vi "test.vi"() -> ()   [LabVIEW 2010]
uses:
  XIntensityCompensation.xctl
panel:
  in  "free-run mode?":bool
  in  "stop":bool
  in  "XIntensityCompensation":cluster{"A":dbl, "lambda":dbl[unit], "C":dbl}(xcontrol)
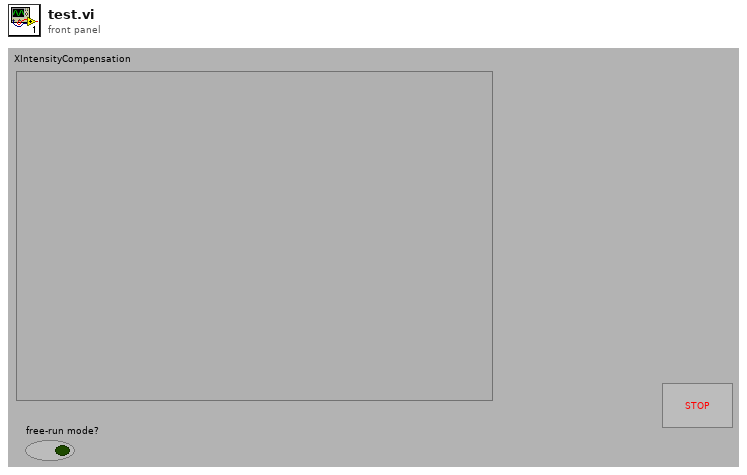
[diagram p1: front panel]
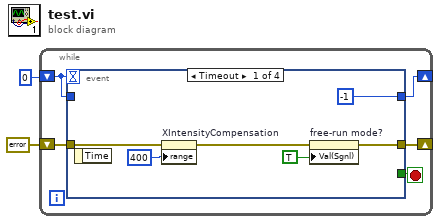
[diagram p0: block diagram]
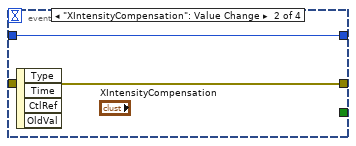
[diagram p2: hidden frame]
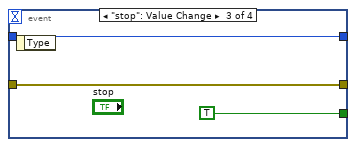
[diagram p3: hidden frame]
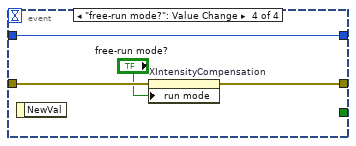
[diagram p4: hidden frame]
diagram:
  n1 = while {
    shift-right: [w5] -> _
    shift-left: errorcluster {"status"=FALSE, "code"=0, "source"=""} ("error in (no error)") -> [w6]
    shift-right: [w3] -> _
    shift-left: 0 -> [w4]
    stop <- w7 stop-if-true
    n2 = event shown="[0] Timeout" {
      selector: _ -> [_ _ _ _]
      dyn-events: _ -> [_ _ _ _]
      timeout: w4 -> [_ _ _ _]
      tunnel: [_ _ TRUE _] -> w7
      tunnel: w6 -> [w10 w15 w17 w22]
      tunnel: [w12 w15 w17 w21] -> w5
      tunnel: w4 -> [_ w14 w16 w20]
      tunnel: [-1 w14 w16 w20] -> w3
      event Timeout {
        n3 = event-data() -> ()  [unwired: 1 in, 1 out]
        n4 = property on="XIntensityCompensation" class="XIntensityCompensation (strict)"(error in=w10, "range"=400) -> (error out=w8:errorcluster)  [unwired: 1 in, 1 out]
        n5 = property on="free-run mode?" class="Bool (strict)"(error in=w8, "Val(Sgnl)"=TRUE ("Value (Signaling)")) -> (error out=w12:errorcluster)  [unwired: 1 in, 1 out]
      }
      event "XIntensityCompensation": Value Change {
        n6 = event-data() -> ()  [unwired: 1 in, 4 out]
      }
      event "stop": Value Change {
        n7 = event-data() -> ()  [unwired: 1 in, 1 out]
      }
      event "free-run mode?": Value Change {
        n8 = event-data() -> ()  [unwired: 1 in, 1 out]
        n9 = property on="XIntensityCompensation" class="XIntensityCompensation (strict)"(error in=w22, "run mode"="free-run mode?") -> (error out=w21:errorcluster)  [unwired: 1 in, 1 out]
      }
    }
  }
